vi "RangeToColor.vi"(9 "Really Close (in)":dbl, 10 "Close (in)":dbl, 11 "Range (in)":dbl) -> (2 "Range Color":u32(colorbox))   [LabVIEW 2018]
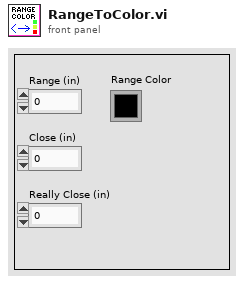
[diagram p1: front panel]
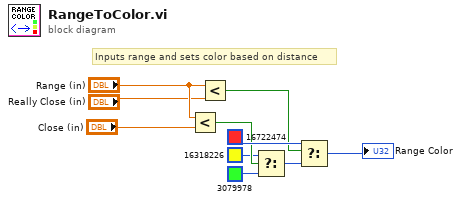
[diagram p0: block diagram]
diagram:
  # "Inputs range and sets color based on distance"
  n1 = Less?(x="Range (in)", y="Close (in)") -> (x < y?=w5:bool)
  n2 = Less?(x="Range (in)", y="Really Close (in)") -> (x < y?=w7:bool)
  n3 = Select(t=u32 16318226 ("Color Box"), s=w5, f=u32 3079978 ("Color Box")) -> (s? t:f=w8:u32)
  n4 = Select(t=u32 16722474 ("Color Box"), s=w7, f=w8) -> (s? t:f=→"Range Color":u32)
